vi "Actor Core.vi"(8 "error in":errorcluster, 11 "TDMS Data Logger Actor in":refnum<class "TDMS Data Logger Actor.lvclass">) -> (0 "error out":errorcluster, 3 "Actor out":refnum<class "Actor.lvclass">)   [LabVIEW 2024, in "TDMS Data Logger Actor.lvlib" / "TDMS Data Logger Actor.lvclass"]
doc: "<p>(<strong>Filename</strong>: <span class=\"dnl\">Actor Framework.lvlib:Actor.lvclass:Actor Core.vi</span>)</p>\n<p>Receives messages to the actor, reacts to them, and initiates any error handling that may shut the actor down.</p>\n<p>Descendant classes may override this VI to append parallel tasks for the actor to complete while it handles messages. Overrides use the <a href=\"nihelplauncher://docs/csh?context=lvcore_glang_udclass\">Call Parent Class Method</a> node.</p>"
uses:
  TDMS Data Logger Actor.lvclass
  <vilib>/ActorFramework/Actor/Actor.lvclass
  TDMS Data Logger Actor Messages/Write Data Msg/Write Data Msg.lvclass
  <vilib>/ActorFramework/Actor/Actor.lvclass/Actor.ctl
  <vilib>/ActorFramework/Message Enqueuer/Message Enqueuer.lvclass/Message Enqueuer.ctl
  <vilib>/ActorFramework/Message Enqueuer/Init from Existing Queue.vi
  <vilib>/ActorFramework/Message Enqueuer/Message Enqueuer.lvclass
  TDMS Data Logger Actor.lvclass/TDMS Data Logger Actor.ctl
  C:/Program Files (x86)/National Instruments/LabVIEW 2024/vi.lib/ActorFramework/Actor/Actor.lvclass
  C:/Users/uspoaotto/OneDrive - Oregon Tool/Desktop/working copies/dataLogger/TDMS Data Logger Actor/TDMS Data Logger Actor/TDMS Data Logger Actor.lvclass
  C:/Users/uspoaotto/OneDrive - Oregon Tool/Desktop/working copies/dataLogger/Data Logger Actor Interface/Data Logger Actor Interface/Data Logger Actor Interface.lvclass
  C:/Program Files (x86)/National Instruments/LabVIEW 2024/vi.lib/ActorFramework/Message/Message.lvclass
  C:/Users/uspoaotto/OneDrive - Oregon Tool/Desktop/working copies/dataLogger/TDMS Data Logger Actor/TDMS Data Logger Actor Messages/Write Data Msg/Write Data Msg.lvclass
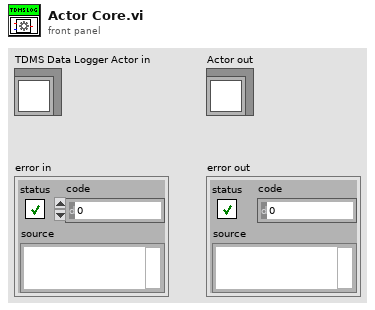
[diagram p1: front panel]
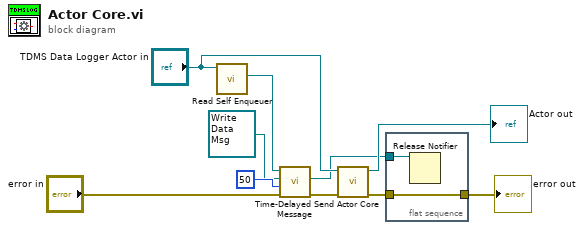
[diagram p0: block diagram]
diagram:
  n1 = call <vilib>:"Read Self Enqueuer.vi"("Actor"="TDMS Data Logger Actor in") -> ("Self Enqueuer"=w8:refnum<class "Message Enqueuer.lvclass">)  [unwired: 10 in]
  n2 = call <vilib>:"Time-Delayed Send Message.vi"("error in (no error)"="error in", "Milliseconds To Wait"=50, "Message"=refnum<class "Write Data Msg.lvclass"> refnum ("TDMS Data Logger Actor.lvlib:Write Data Msg.lvclass"), "Message Enqueuer"=w8) -> ("error out"=w6:errorcluster, "Delivery Notifier"=w1:refnum<notifier>)  [unwired: 6 in]
  n3 = call-parent "Actor Core.vi"("error in"=w6, "Actor in"="TDMS Data Logger Actor in") -> ("error out"=w3:errorcluster, "Actor out"=→"Actor out":refnum<class "Actor.lvclass">)  [unwired: 8 in]
  n4 = flat-sequence {
    tunnel: w1 -> [w12]
    tunnel: w3 -> [w11]
    tunnel: [w11] -> w2
    frame #0 {
      n5 = Release Notifier(notifier=w12) -> ()  [unwired: 2 in, 3 out]
    }
  }
  "error out" <- w2
